vi "Initialize Subpanel VIs.vi"(8 "error in (no error)":errorcluster) -> (0 "error out":errorcluster, 2 "subpanel to main command event reg":T1, 3 "subpanel info":T2)   [LabVIEW 2017, in "NI_Robotics_Configure Steering Frame.lvlib"]
uses:
  <vilib>/robotics/Dialog/Configure Steering Frame/NI_Robotics_Configure Steering Frame.lvlib
  <vilib>/robotics/Dialog/Configure Steering Frame/Subpanel Info.ctl
  <vilib>/robotics/Dialog/Configure Steering Frame/Main to Subpanel Command Event.ctl
  <vilib>/robotics/Dialog/Configure Steering Frame/Main to Subpanel Command.ctl
  <vilib>/robotics/Steering/Steering Frame/NI_Robotics_Steering Frame.lvclass
  <vilib>/robotics/Dialog/Configure Steering Frame/Subpanel to Main Command Event Reg.ctl
  <vilib>/robotics/Dialog/Configure Steering Frame/User Defined Frame Subpanel/User Defined Frame Subpanel.lvlib
  <vilib>/robotics/Dialog/Configure Steering Frame/Differential Frame Subpanel/Differential Frame Subpanel.lvlib
  <vilib>/robotics/Dialog/Configure Steering Frame/Ackermann Frame Subpanel/Ackermann Frame Subpanel.lvlib
  <vilib>/robotics/Dialog/Configure Steering Frame/Mecanum Frame Subpanel/Mecanum Frame Subpanel.lvlib
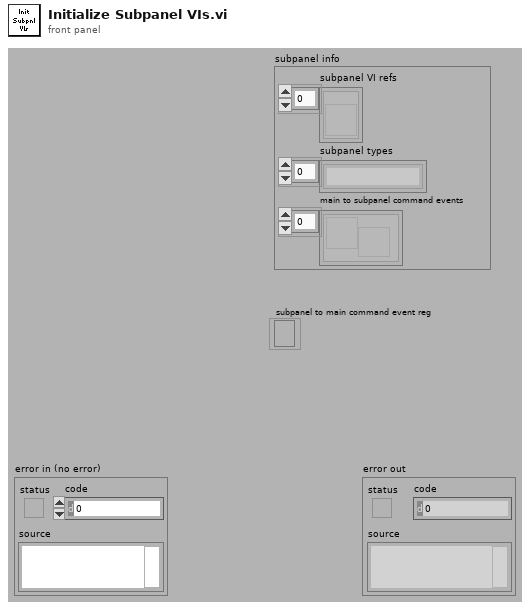
[diagram p1: front panel]
types:
  T1 = typedef "NI_Robotics_Configure Steering Frame.lvlib/Subpanel to Main Command Event Reg.ctl" = refnum<event-registration>
  T2 = typedef "NI_Robotics_Configure Steering Frame.lvlib/Subpanel Info.ctl" = cluster{"subpanel VI refs":refnum<vi>[], "subpanel types":string[], "main to subpanel command events":T3[]}
  T3 = typedef "NI_Robotics_Configure Steering Frame.lvlib/Main to Subpanel Command Event.ctl" = refnum<user-event>
  T4 = typedef "NI_Robotics_Configure Steering Frame.lvlib/Subpanel to Main Command Event.ctl" = refnum<user-event>
  T5 = typedef "NI_Robotics_Configure Steering Frame.lvlib/Main to Subpanel Command Event Reg.ctl" = refnum<event-registration>
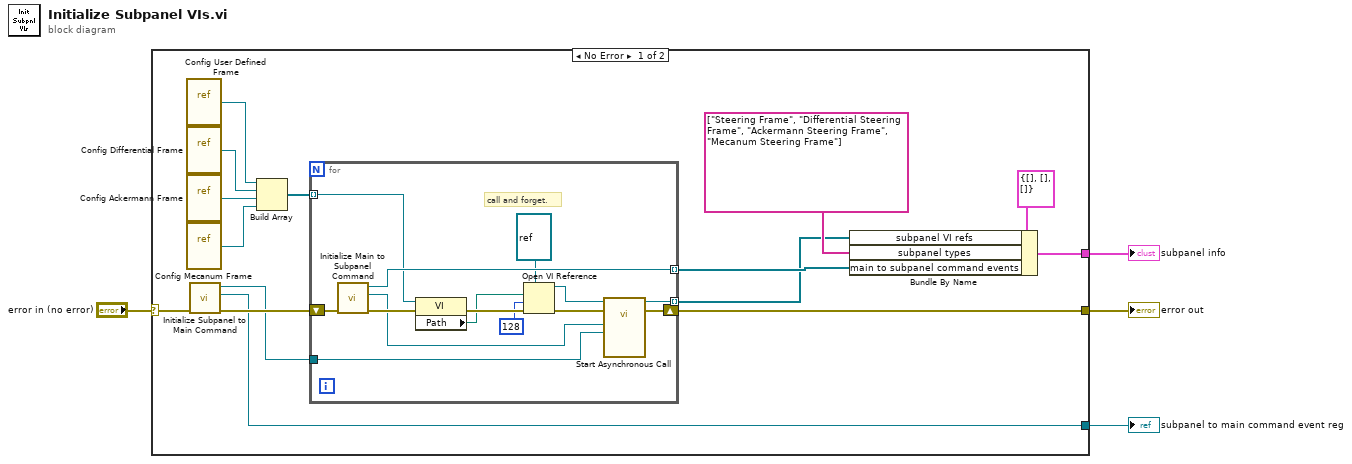
[diagram p0: block diagram]
diagram:
  n1 = case shown="No Error" "error in (no error)" {
    selector: "error in (no error)" -> [w12 w34]
    tunnel: [w15 w34] -> w4
    tunnel: [w14 _] -> w3
    tunnel: [w13 _] -> w2
    frame No Error {
      n2 = vi-ref <vilib>:"Config User Defined Frame.vi"() -> (w11:refnum<vi>)
      n3 = vi-ref <vilib>:"Config Differential Frame.vi"() -> (w10:refnum<vi>)
      n4 = vi-ref <vilib>:"Config Ackermann Frame.vi"() -> (w9:refnum<vi>)
      n5 = vi-ref <vilib>:"Config Mecanum Frame.vi"() -> (w8:refnum<vi>)
      n6 = call <vilib>:"Initialize Subpanel to Main Command.vi"("error in (no error)"=w12) -> ("error out"=w19:errorcluster, "subpanel to main command event reg"=w13:T1, "subpanel to main command event"=w7:T4)  [unwired: 8 in]
      n7 = Build Array(w11, w10, w9, w8) -> (w6:refnum<vi>[])
      n8 = for {
        tunnel: w6 -> [w27] mode=indexing
        tunnel: w7 -> [w30]
        tunnel: [w29] -> w16 mode=indexing
        shift-right: [w28] -> w15
        shift-left: w19 -> [w33]
        tunnel: [w26] -> w5 mode=indexing
        # "call and forget."
        n9 = call <vilib>:"Initialize Main to Subpanel Command.vi"("error in (no error)"=w33) -> ("error out"=w32:errorcluster, "main to subpanel command event reg"=w31:T5, "main to subpanel command event"=w29:T3)  [unwired: 8 in]
        n10 = property class="VI"(reference=w27, error in=w32) -> (error out=w25:errorcluster, "Path"=w24:path)  [unwired: 1 out]
        n11 = Open VI Reference(type specifier VI Refnum (for type only)=refnum<vi> refnum, vi path=w24, options=128, error in (no error)=w25) -> (vi reference=w22:refnum<vi>, error out=w21:errorcluster)  [unwired: 2 in]
        n12 = call-by-ref "Start Asynchronous Call"(reference=w22, error in=w21, "subpanel to main command event"=w30, "main to subpanel command event reg"=w31) -> (reference out=w26:refnum<vi>, error out=w28:errorcluster)  [unwired: 10 in]
      }
      n13 = Bundle By Name(cluster=T2 {"subpanel VI refs"=[], "subpanel types"=[], "main to subpanel command events"=[]} ("subpanel info"), "subpanel VI refs"=w5, "subpanel types"=string[] ["Steering Frame", "Differential Steering Frame", "Ackermann Steering Frame", "Mecanum Steering Frame"] ("wheel types"), "main to subpanel command events"=w16) -> (w14:T2)
    }
    frame Error {
    }
  }
  "error out" <- w4
  "subpanel info" <- w3
  "subpanel to main command event reg" <- w2
